vi "Create HTML.vi"(7 "FP Reference":refnum<class "Web Front Panel.lvclass">, 8 "error in (no error)":errorcluster, 10 "VI Identifier":string, 11 "Graph In":refnum<class "Graph.lvclass">) -> (0 "error out":errorcluster, 1 "js code for controls":string, 2 "js variables":string, 3 "Graph Out":refnum<class "Graph.lvclass">, 4 "script dependencies":string[](array[string]), 5 "HTML":string, 6 "js code for indicators":string)   [LabVIEW 2017, in "Front Panel Publisher.lvlib" / "Graph.lvclass"]
uses:
  Graph.lvclass
  Object_class/Object.lvclass
  Control_class/Control.lvclass
  Front Panel Publisher.lvlib
  Web Front Panel_class/Web Front Panel.lvclass
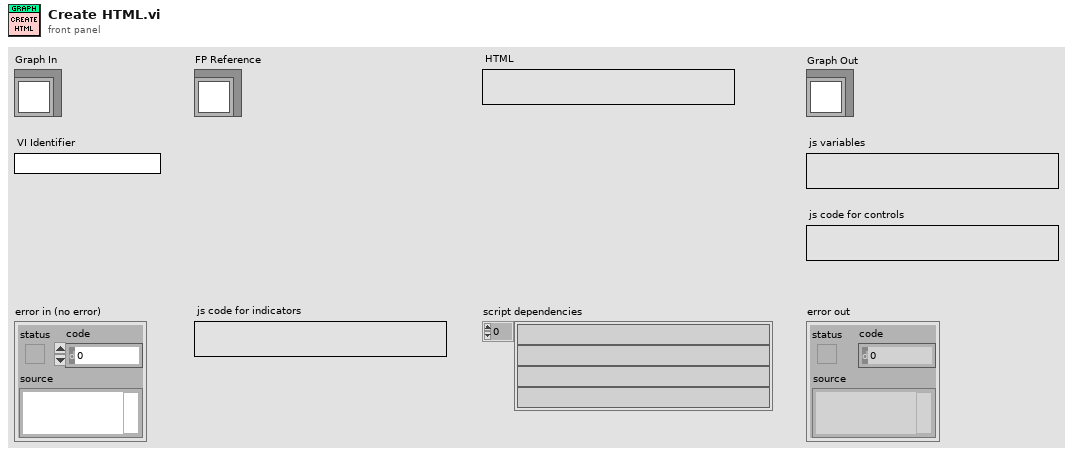
[diagram p1: front panel]
types:
  T1 = typedef "Front Panel Publisher.lvlib/Object.lvclass/Attributes.ctl" = cluster{"UID":i32, "Type":string, "Starting Location":T2, "Reference":refnum<vi>, "Cluster Component":bool, "Starting Rect Position":cluster{"Left":i16, "Top":i16}, "Owning Pane":refnum<vi>, "Master Total Rect Delta":T3}
  T2 = typedef "Front Panel Publisher.lvlib/Object.lvclass/Coordinates.ctl" = cluster{"Left":i32, "Top":i32, "Height":u32, "Width":u32}
  T3 = typedef "LVRectTypeDef.ctl" = cluster{"Left":i16, "Top":i16, "Right":i16, "Bottom":i16}
  T4 = typedef "Front Panel Publisher.lvlib/Control.lvclass/Attributes.ctl" = cluster{"Description":string, "Indicator":bool, "Default Value":variant, "Control Index":i32, "Label":refnum<class "Text.lvclass">, "Caption":refnum<class "Text.lvclass">, "Image b64":string, "No Control Index":bool, "Display Mode":T5}
  T5 = typedef "Front Panel Publisher.lvlib/Web Front Panel.lvclass/Enum - Control Display Mode.ctl" = enum16{"Value Only", "Value and Visibility", "Boolean Value Only", "Boolean Value and Visibility", "Control is Image", "Image and Visibility"}
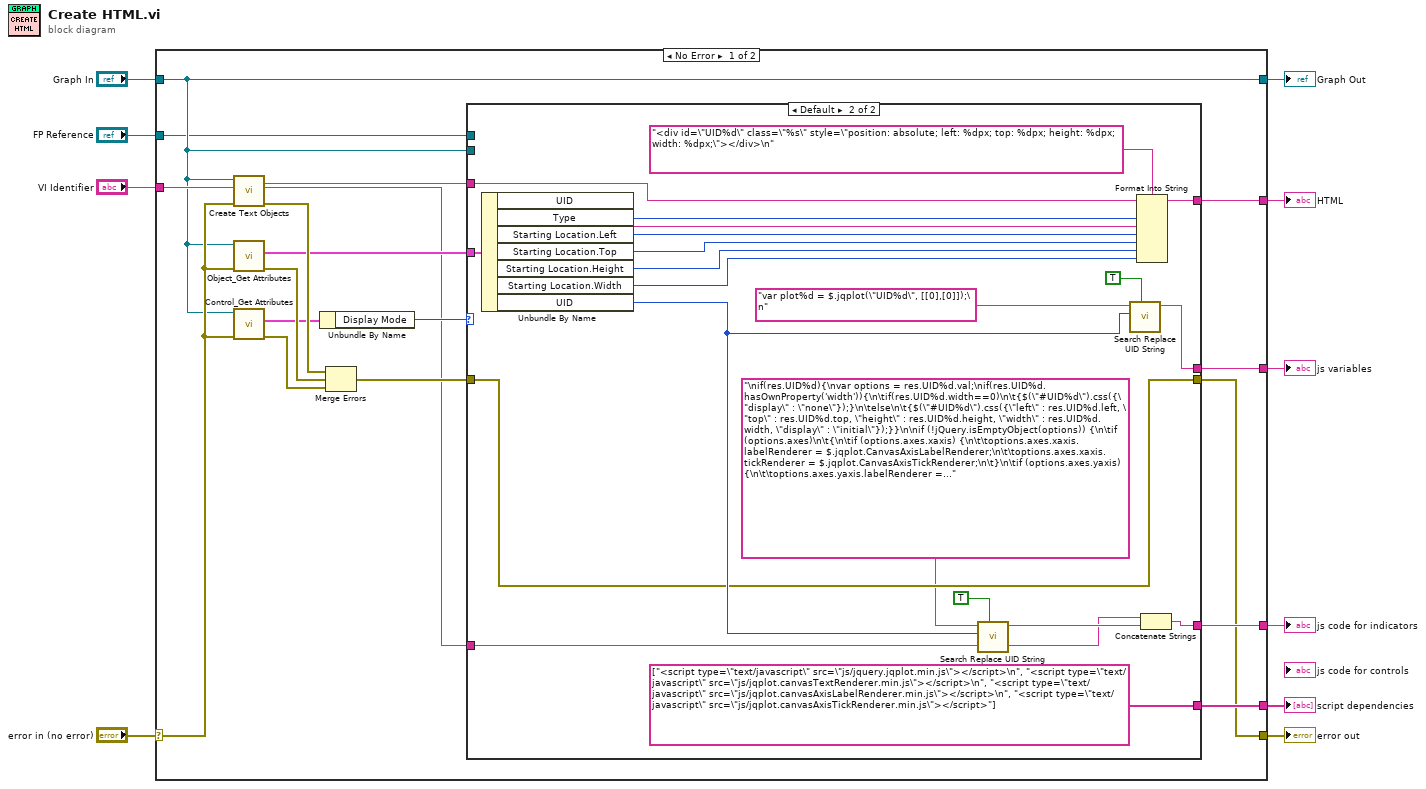
[diagram p0: block diagram]
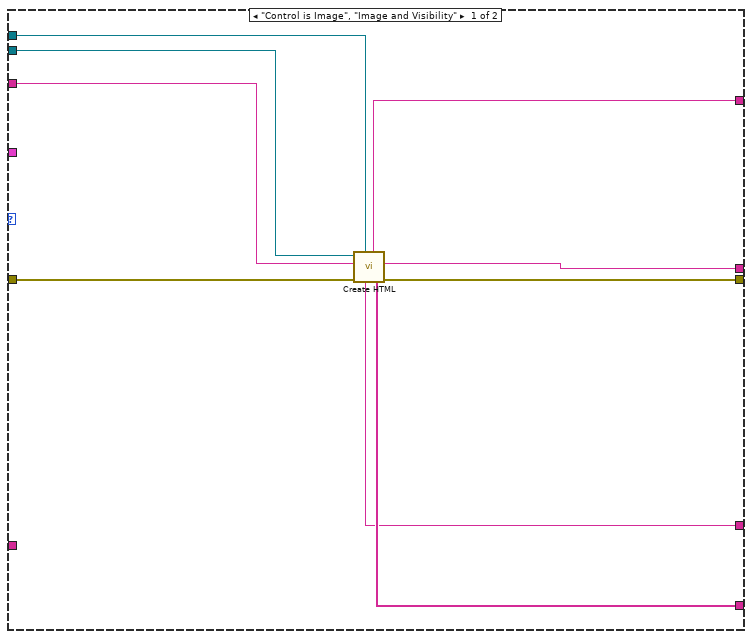
[diagram p2: hidden frame]
diagram:
  n1 = case shown="No Error" "error in (no error)" {
    selector: "error in (no error)" -> [w26 w60]
    tunnel: [w13 w60] -> w9
    tunnel: [w24 _] -> w8
    tunnel: [w19 _] -> w7
    tunnel: [w18 _] -> w6
    tunnel: [w22 _] -> w5
    tunnel: "VI Identifier" -> [w20 _]
    tunnel: [w14 w59] -> w3
    tunnel: "Graph In" -> [w14 w59]
    tunnel: "FP Reference" -> [w11 _]
    frame No Error {
      n2 = call-dynamic "Create Text Objects.vi"("error in (no error)"=w26, "VI Name"=w20, "Control In"=w14) -> ("error out"=w27:errorcluster, "JS Indicator"=w12:string, "HTML"=w21:string)  [unwired: 5 in, 1 out]
      n3 = call "Object_Get Attributes.vi"("error in (no error)"=w26, "Object In"=w14) -> ("error out"=w28:errorcluster, "Object Attributes"=w23:T1)  [unwired: 7 in, 1 out]
      n4 = call "Control_Get Attributes.vi"("error in (no error)"=w26, "Control In"=w14) -> ("error out"=w25:errorcluster, "Control Attributes"=w16:T4)  [unwired: 7 in, 1 out]
      n5 = Unbundle By Name(w16) -> ("Display Mode"=w17:T5)
      n6 = Merge Errors(w27, w28, w25) -> (w15:errorcluster)
      n7 = case shown="Default" w17 {
        tunnel: [w34 w51] -> w24
        tunnel: w23 -> [_ w50]
        tunnel: [w32 string[] ["<script type=\"text/javascript\" src=\"js/jquery.jqplot.min.js\"></script>\n", "<script type=\"text/javascript\" src=\"js/jqplot.canvasTextRenderer.min.js\"></script>\n", "<script type=\"text/javascript\" src=\"js/jqplot.canvasAxisLabelRenderer.min.js\"></script>\n", "<script type=\"text/javascript\" src=\"js/jqplot.canvasAxisTickRenderer.min.js\"></script>"]] -> w22
        tunnel: w21 -> [w36 w48]
        tunnel: [w33 w44] -> w19
        tunnel: [w30 w40] -> w18
        tunnel: w15 -> [w35 w41]
        tunnel: w14 -> [w37 _]
        tunnel: [w31 w41] -> w13
        tunnel: w12 -> [_ w39]
        tunnel: w11 -> [w29 _]
        frame "Control is Image", "Image and Visibility" {
          n8 = call-parent "Create HTML.vi"("FP Reference"=w29, "error in (no error)"=w35, "VI Identifier"=w36, "Control In"=w37) -> ("error out"=w31:errorcluster, "js variables"=w33:string, "script dependencies"=w32:string[], "HTML"=w34:string, "js code for indicators"=w30:string)  [unwired: 1 in, 2 out]
        }
        frame Default {
          n9 = Unbundle By Name(w50) -> ("UID"=w57:i32, "Type"=w56:string, "Starting Location.Left"=w55:i32, "Starting Location.Top"=w54:i32, "Starting Location.Height"=w53:u32, "Starting Location.Width"=w52:u32, "UID"=w43:i32)
          n10 = call "Search Replace UID String.vi"("Replace All Numeric Inputs"=TRUE, "UID"=w43, "Input String"="\nif(res.UID%d){\nvar options = res.UID%d.val;\nif(res.UID%d.hasOwnProperty('width')){\n\tif(res.UID%d.width==0)\n\t{$(\"#UID%d\").css({\"display\" : \"none\"});}\n\telse\n\t{$(\"#UID%d\").css({\"left\" : res.UID%d.left, \"top\" : res.UID%d.top, \"height\" : res.UID%d.height, \"width\" : res.UID%d.width, \"display\" : \"initial\"});}}\n\nif (!jQuery.isEmptyObject(options)) {\n\tif (options.axes)\n\t{\n\tif (options.axes.xaxis) {\n\t\toptions.axes.xaxis.labelRenderer = $.jqplot.CanvasAxisLabelRenderer;\n\t\toptions.axes.xaxis.tickRenderer = $.jqplot.CanvasAxisTickRenderer;\n\t}\n\tif (options.axes.yaxis) {\n\t\toptions.axes.yaxis.labelRenderer = $.jqplot.CanvasAxisLabelRenderer;\n\t\toptions.axes.yaxis.tickRenderer = $.jqplot.CanvasAxisTickRenderer;\n\t}\n\tif (options.axes.y2axis) {\n\t\toptions.axes.y2axis.labelRenderer = $.jqplot.CanvasAxisLabelRenderer;\n\t\toptions.axes.y2axis.tickRenderer = $.jqplot.CanvasAxisTickRenderer;\n\t}\n\t}\n\tplot%d.replot(options);\n}}\n") -> ("Output String"=w47:string)  [unwired: 8 in]
          n11 = call "Search Replace UID String.vi"("Replace All Numeric Inputs"=TRUE, "UID"=w43, "Input String"="var plot%d = $.jqplot(\"UID%d\", [[0],[0]]);\n") -> ("Output String"=w44:string)  [unwired: 8 in]
          n12 = Format Into String(format string="<div id=\"UID%d\" class=\"%s\" style=\"position: absolute; left: %dpx; top: %dpx; height: %dpx; width: %dpx;\"></div>\n", initial string=w48, w57, w56, w55, w54, w53, w52) -> (resulting string=w51:string)  [unwired: 1 in, 1 out]
          n13 = Concatenate Strings(w39, w47) -> (w40:string)
        }
      }
    }
    frame Error {
    }
  }
  "error out" <- w9
  "Graph Out" <- w3
  "HTML" <- w8
  "js variables" <- w7
  "script dependencies" <- w5
  "js code for indicators" <- w6
